vi "gfitsio-create-tbl.vi"(4 "tbltype":T1 items=["ANY_HDU"=-1, "IMAGE_HDU"=0, "ASCII_TBL"=1, "BINARY_TBL"=2], 7 "extname":string, 8 "error in (no error)":errorcluster, 11 "gfits refnum":T2) -> (0 "error out":errorcluster, 3 "dup gfits refnum":T2)   [LabVIEW 2011, in "gfitsio.lvlib"]
doc: "Create a new ASCII or bintable table extension. If the FITS file is currently empty then a dummy primary array will be created before appending the table extension to it. The tbltype parameter defines the type of table and can have values of ASCII_TBL or BINARY_TBL. The naxis2 parameter gives the initial number of rows to be created in the table, and should normally be set = 0. CFITSIO will automatically increase the size of the table as additional rows are written. A non-zero number of rows may be specified to reserve space for that many rows, even if a fewer number of rows will be written. The tunit and extname parameters are optional and a null pointer may be given if they are not defined. The FITS Standard recommends that only letters, digits, and the underscore character be used in column names (the ttype parameter) with no embedded spaces. Trailing blank characters are not significant. It is recommended that all the column names in a given table be unique within the first 8 characters, and strongly recommended that the names be unique within the first 16 characters."
uses:
  gfitsio.lvlib
  gfitsio-refnum.ctl
  cfitsio-hdutypes.ctl
  gfitsio.dll
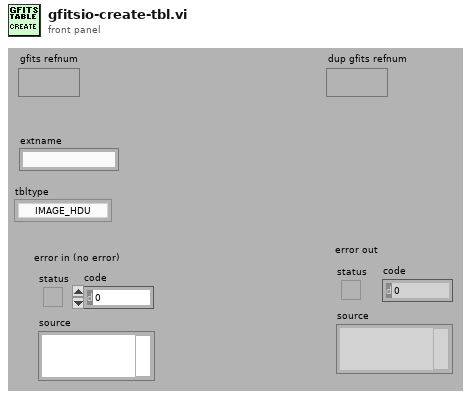
[diagram p1: front panel]
types:
  T1 = typedef "gfitsio.lvlib/cfitsio-hdutypes.ctl" = i32
  T2 = typedef "gfitsio.lvlib/gfitsio-refnum.ctl" = refnum<k1>
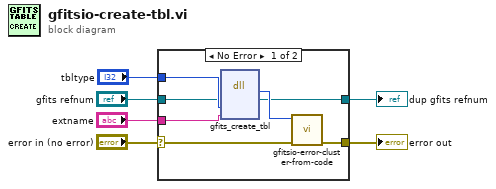
[diagram p0: block diagram]
diagram:
  n1 = case shown="No Error" "error in (no error)" {
    selector: "error in (no error)" -> [w11 w15]
    tunnel: [w13 w15] -> w6
    tunnel: "extname" -> [w10 _]
    tunnel: "gfits refnum" -> [w7 w14]
    tunnel: [w8 w14] -> w3
    tunnel: "tbltype" -> [w9 _]
    frame No Error {
      n2 = dll-call lib="C:/BonOMM/BonOMM-SAOMM/SubVIs/gfitsio/gfitsio.dll" fn="gfits_create_tbl"("gfits refnum"=w7, "tbltype"=w9, "extname"=w10) -> (w12:i32, "gfits refnum"=w8:T2)  [unwired: 5 in, 2 out]
      n3 = call "gfitsio-error-cluster-from-code.vi"("error in (no error)"=w11, "error code"=w12) -> ("error out"=w13:errorcluster)  [unwired: 9 in]
    }
    frame Error {
    }
  }
  "error out" <- w6
  "dup gfits refnum" <- w3
